vi "Bad Type Error.vi"() -> (0 "Unsupported Type Error":errorcluster)   [LabVIEW 2020, in "G-Embedded-Python-Interpreter-Toolkit.lvlib"]
uses:
  G-Embedded-Python-Interpreter-Toolkit.lvlib
  <vilib>/ErrorRing/Error Ring.xnode
  <vilib>/Utility/error.llb/Error Cluster From Error Code.vi
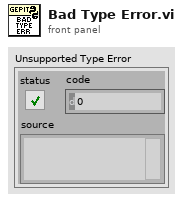
[diagram p1: front panel]
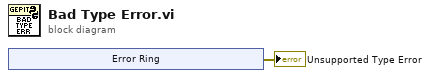
[diagram p0: block diagram]
diagram:
  n1 = xnode "Error Ring"() -> ("error out"=→"Unsupported Type Error":errorcluster)
